vi "Error Message.vi"(10 "Error Code":i32) -> (2 "Error Message":string)   [LabVIEW 2019, in "Andeen-Hagerling 2700(400 firmware).lvlib"]
doc: "This VI converts a numeric error code from the bridge to an english error message."
uses:
  Andeen-Hagerling 2700(400 firmware).lvlib
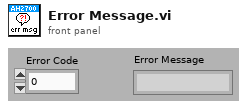
[diagram p1: front panel]
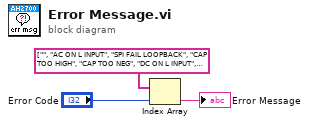
[diagram p0: block diagram]
diagram:
  n1 = Index Array(array=string[] ["", "AC ON L INPUT", "SPI FAIL LOOPBACK", "CAP TOO HIGH", "CAP TOO NEG", "DC ON L INPUT", "ERRATIC INPUT", "EXCESS NOISE", "", "H TO GND SHORT", "H TO L SHORT", "INDETERM OFFSCALE", "L TO GND SHORT", "LOSS TOO HIGH", "LOSS TOO NEG", "OVEN NOT READY", "VOLTAGE REDUCED", "BUTTON BUF FULL", "AMBIGUOUS WORD: ", "BAD PARAMETER", "BAD PASSCODE", "CAL DATA ABSENT", "WRONG BANK", "CAL DATA ERROR 0", "CAL DATA ERROR 1", "CAL DATA ERROR 2", "CAL DATA ERROR 3", "CAL DATA ERROR 4", "CMD NOT OPERABLE", "EXTERNAL TRIGGER", "EEPROM ERROR", "FILE NOT FOUND", "GPIB OUTBUF FULL", "ILLEGAL WORD: ", "INT CAL FAILURE", "OUT OF SPACE", "MACRO NEST ERROR", "SYNTAX ERROR", "BAD PARAMETER: ", "UPDATE STD ERROR", "LINE TOO LONG", "ARE YOU SURE?", "CAL CODE>", "CALIBRATE BUSY", "CONN DC TO BIAS >", "CONN PI HI TO LO >", "CONN TER TO HIGH >", "DEVICE CLEAR\n>", "", "DISCONN SETUP >", "LOCAL LOCKOUT", "ONR CODE>", "PASSCODE>", "READ LO <0.02V >", "READ LO 100V >", "READ VLT FOR R603 >", "READ VLT FOR R604", "RPL CODE>", "SHORT LO TO GND >", "USER CODE>", "READY>", "", "READY\n>", "", "READY MC#", "", "READY MC\n#", "", "RESET", "", "READY DV @", "", "READY DV\n@", "", "+", "", "", "", "CHECKSUM ERROR U306", "CHECKSUM ERROR U307", "CPU TEST PASSED", "DUAL ADR ERROR", "EEPROM SAFE ERR", "FREQ RATIO ERROR", "GPIB ERROR", "HI RAM ERROR ", "INTERRUPT ERROR", "UART ERROR", "", "", "WAIT FOR DEV ERROR", "WAITFOR EXTERNAL", "OFF", "ON", "AUTO", "PASS", "FAIL", "SCOPE ", " FUNC", " ANLG", "ZERO", "BASIC", "GAUGE", "SERIAL", "GPIB", "MACRO", "DEV", "SCAN", "BIGGEST CHANGE", "C", "CAP ", "INT", "LAST", "FACT ", "UPDT ", "PPM", "", "TRF", "USER CAP", "", ">", "=", " BWDECIMAL", "PCT%", "", "P%", "", "R", "Z", "NS", "DF", "KO", "GP", "JP", "VIDEO", "PRINTER", "BUSY", "DOWNLOAD DONE OK", " NO DATA", " DID NOT FINISH", "BAD DATA", "FLASH ERROR", "GO TO ROM BANK", "EMPTY OR BAD BANK", "READY BANK ROM", "", "BANK ROM", "", "BANK ROM", "", "RTC WAS RESET ", "", "RTC WAS RESET", "", "RTC WAS RESET", "", "CAL DATA ERROR 5", "CAL DATA ERROR 6", "CAL DATA ERROR 7", "CAL DATA ERROR 8", "CAP DEV TOO LOW", "CAP DEV TOO HIGH", "LOSS DEV TOO LOW", "LOSS DEV TOO HIGH", "DEV ERRATIC", "PREAMP OVERLOAD", "DEV CONFLICT", "UNITS CONFLICT", "ZERO CONFLICT", "DEV INIT FAILURE", "MODE TOO BIG", "EACH", "INNER", "SECOND", "THIRD", "DEVICE CLEAR", "", "DISCRETE", " LOG10", " LOG2", "LINEAR", "DIRECTION", "PERDECADE", "PEROCTAVE", "V", "HZ", "METHOD CONFLICT", "FLOOR CEILING INVALID", "NO COUPLED PARAMETERS", "COUNT MAX REACHED", "GROUND ", "BIAS", "DEV", "NO ERROR FOUND", "NO DATA FOUND", "OLD CAL OK?", "", "DEV SPAN TOO BIG", "ERROR", "NORMAL", "CAP DEV ERRATIC", "LOSS DEV ERRATIC", "ABOUNDS REVERSAL", "LIMITS REVERSAL", "NONE", "ODD", "EVEN", "FLOATING", "SCIENTIFIC", "ENGINEERING", "VARIABLE", "FIXED", "OFF", "ILOW", "IHIGH", "OFF", "LINE_REJ", "ASYNC", " INACTIVE", " ACTIVE", "SERIAL", "ROM", "FLASH1", "FLASH2", "UNLIMITED", "CAL DATA ERROR 9", "", "", "SCOPE", "ERROR", "SUMMARY", "ALL", "OFF", "READINGS", "RESULTS", "CMDS_TOO", "GIVE_ERR", "BUFFER", "TALKONLY", "PRI_ONLY", "PNSCNDRY", "NUMERIC", "ENGLISH", "NOT FOUND", "CR_LF", "SEMICOLON", "ZERO FREQ MISMATCH", "TEMP OUT OF RANGE", "CAL PAST DUE", "CALI TEMP CHANGED", "INT", "CAP", "TRF", "CABLE", "DCXTPG1", "TTA1"] ("subarray"), index="Error Code") -> (element=→"Error Message":string)
